vi "Send_SET_8Bits.vi"(8 "error in (no error)":errorcluster, 10 "Channel":u8, 11 "NXP in":refnum<class "NXP.lvclass">) -> (0 "error out":errorcluster, 2 "Response":string, 3 "NXP out":refnum<class "NXP.lvclass">)   [LabVIEW 2019, in "NXP.lvclass"]
uses:
  NXP.lvclass
  Clase Padre/Serial Device.lvclass
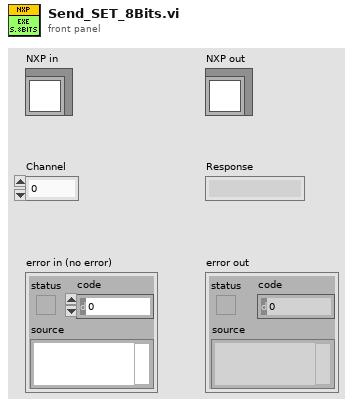
[diagram p1: front panel]
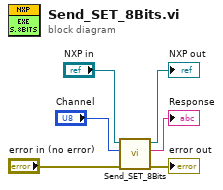
[diagram p0: block diagram]
diagram:
  n1 = call-parent "Send_SET_8Bits.vi"("error in (no error)"="error in (no error)", "Channel"="Channel", "Serial Device in"="NXP in") -> ("error out"=→"error out":errorcluster, "Response"=→"Response":string, "Serial Device out"=→"NXP out":refnum<class "NXP.lvclass">)  [unwired: 6 in]
